vi "UHR-Fleezers Control (host) - Lorentz v3.vi"() -> ()   [LabVIEW 2014] (continued)
  in  "Red FB Gains":T14={"proportional gain (Kc)"=10, "integral gain (Kc*Ts/Ti)"=5, "derivative gain (Kc*Td/Ts)"=0}
  in  "Phase adj. (RI)":i16=20
  out "RI relative phase":i16
  in  "+ phase (RI)":bool
  in  "- phase (RI)":bool
  in  "Blue Laser Modulation Mode":string(combo)
  out "Digital Modulation":bool
  out "Analog Modulation":bool
  out "Laser On":bool
  in  "Get Blue Laser State":bool
  out "Blue laser intensity (V)":dbl
  out "Relative phase (BI AO)":i16
  out "Relative phase (BI DO)":i16
  out "Late Counter (BI DO)":u8
  out "Late Counter (BI AO)":u8
  in  "Initial Phase Adjustment (BI DO)":i16=65
  in  "Initial Phase Adjustment (BI AO)":i16
  in  "Phase adj. (BI AO)":i16=20
  in  "+ phase (BI AO)":bool
  in  "- phase (BI AO)":bool
  in  "Blue int AO ON count adjust":u16=150
  in  "Blue FB Gains":T14={"proportional gain (Kc)"=10, "integral gain (Kc*Ts/Ti)"=5, "derivative gain (Kc*Td/Ts)"=0}
  in  "- phase (BI DO)":bool
  in  "+ phase (BI DO)":bool
  in  "Phase adj. (BI DO)":i16=20
  out "Blue AI Count":u16=600
  in  "Delay (ms)":i32=500
  in  "Send string\nto Blue Laser":bool
  in  "command string":string
  out "command string sent":string="sames 0"
  out "read blue buffer":string
  out "Blue Error Out":errorcluster={"status"=TRUE, "code"=-1073807346, "source"="VISA Write in serial write macro.vi->UHR-Fleezers Control (host) - Lorentz v3.vi"}
  in  "VISA resource name":refnum<visa-resource-name>="Blue-Laser-COM7"
  in  "Blue Laser Modulation\nPower (mW)":string="80"
  in  "Blue Laser Power (mW)\n(Constant Power Mode)":string="70"
  out "Serial Error out":errorcluster={"status"=FALSE, "code"=1073676294, "source"="VISA Read in Arduino input-output.vi->UHR-Fleezers Control (host) - Lorentz v3.vi"}
  in  "PSD Data Period (s)":dbl=0.02 caption="PSD data period (s)" format="%#_6p"
  in  "Flip X Sign":bool=TRUE
  in  "Trap Position FIFO Depth":u32=300000 format="%.0p"
  in  "# Samples/trap":u32=20000
  out "Trap AI Elements/DMA read":u32=320000 format="%.0p"
  out "Ave. Rate (Hz)":dbl=200000.0 format="%#_6p"
  out "FIFO El. Rem.":u32 format="%.0p"
  in  "Phase adj. (AI1)":i16=10
  out "Relative phase (AI1)":i16=-170
  in  "+ phase (AI1)":bool
  in  "- phase (AI1)":bool
  out "Late Counter (AI1)":u8
  in  "Initial Phase Adjustment (AI1)":i16=170
  out "AI rate (Hz)":dbl=200000.0 format="%#_6p"
  in  "AI Count (ticks)":u16=200
  out "# Samples/channel":u32=40000 format="%.0p"
  in  "Trap AI FIFO Depth":u32=900000
  in  "Detector Type":string(combo)="IR-QPD + PSD + FB-QPD X position"
  in  "N Acq Sets (Traps + Fl.)":i16=3
  in  "Sets to FIFO (Traps)":T22={"Set 1"=TRUE, "Set 2"=TRUE, "Set 3"=FALSE}
  in  "FPGA Ave.":dbl=1.0 min=1.0 step=1.0
  out "Ave. Period (s)":dbl=5e-06 format="%#_6p"
  out "DMA Update Period (s)":dbl=0.3
  out "FPGA Averaging":bool
  out "Trap Sets":u32=2
  out "Counts/DMA":dbl=12000000.0 format="%#_6p"
  out "Trap Pos FIFO El Remaining":u32=3 format="%.0p"
  out "Trap Pos Elements/DMA read":u32=200000 format="%.0p"
  out "Trap AI FIFO Timeout":u16=1256
  out "Trap Pos FIFO Timeout":u16=10635
  in  "Serial Settings for arduino":T23={"baud rate"=9600, "data bits"=8, "parity"=enum."None", "stop bits"=10, "flow control"=0, "Time out (ms)"=1000} {"flow control" items=["None"=0, "XON/XOFF"=1, "RTS/CTS"=2, "DTR/DSR"=4]; "stop bits" items=["1.0"=10, "1.5"=15, "2.0"=20]; "data bits" min=5 max=8 step=1; "baud rate" items=["75"=75, "110"=110, "134"=134, "150"=150, "300"=300, "600"=600, "1200"=1200, "1800"=1800, "2400"=2400, "4800"=4800, "7200"=7200, "9600"=9600, "14400"=14400, "19200"=19200, "28800"=28800, "38400"=38400, "56000"=56000, "57600"=57600, "115200"=115200, "128000"=128000, "230400"=230400]}
  in  "VISA resource name":refnum<visa-resource-name>="COM18"
  in  "Serial Error in":errorcluster
  out "error out":errorcluster
  out "error out 2":errorcluster
  in  "Piezo trap 0 position relative to 75 MHz":cluster{"X (V)":dbl, "Y (V)":dbl}={"X (V)"=3.0, "Y (V)"=0.0}
  in  "Piezo Trap Y cal (nm/V)":dbl=200.0
  in  "Piezo Trap X cal (nm/V)":dbl=200.0
  in  "Bottom  1 Harvard Syringe Pump Serial Port":refnum<visa-resource-name>="Bottom-Pump1-COM5"
  in  "Center Harvard Syringe Pump Serial Port":refnum<visa-resource-name>="Central-Pump2-COM6"
  in  "Lost Tether Alarm Threshold (pN)":dbl=0.5
  in  "AOM X Cal (nm/MHz)":dbl=200.0
  in  "MCL X Cal (nm/V)":dbl=739.5
  out "X RF Amplitude Limits (%)":T24={"Minimum"=0.0, "Maximum"=50.0, "Increment"=1.0}
  out "X RF Frequency Limits (MHz)":T24={"Minimum"=60.0, "Maximum"=90.0, "Increment"=1.0}
  out "Y RF Frequency Limits (MHz)":T24={"Minimum"=0.0, "Maximum"=40.0, "Increment"=0.1}
  out "Y RF Amplitude Limits (%)":T24={"Minimum"=0.0, "Maximum"=45.0, "Increment"=1.0}
  in  "Manip. X?":bool=TRUE
  in  "Manip. Y?":bool
  in  "Force Manip Abort":bool
  out "Read cal error":errorcluster={"status"=TRUE, "code"=7, "source"="Open/Create/Replace File in UHR-Fleezers Control (host) - 15.2.1UCBMengV9.vi<APPEND>\nP:\\Data\\160111\\current.cal"}
  in  "DAQ Delay (ms)":u32=1000
  in  "Start Scan":bool
  in  "Scan axis":bool=TRUE
  in  "Osc. amp. (V)":dbl=5.0
  in  "Osc. center (V)":dbl=5.0
  in  "Osc. freq. (Hz) 2":dbl=1.0
  in  "MCL Mode":u16(ring) items=["Manual Positioning", "Sinusoidal Wave", "Linear Scan"]
  in  "Begin (V)":dbl
  in  "End (V)":dbl=10.0
  in  "N Points":dbl=20.0
  in  "Delay to Interlace (s)":dbl
  in  "Delayed Interlace Start":bool
  in  "Read Lateness and Rel Phase":bool=TRUE
  out "Vec Mean of T1 T2":dbl[](array[numeric])=[nan, nan]
  in  "Cal read wait (s)":u32=5
  out "Time tether formed":timestamp=timestamp(3534521622.0325327 s since 1904-01-01)
  in  "Sample Chamber Stage Serial Port":refnum<visa-resource-name>="Sample-Stage-COM1"
  in  "Chemyx Syringe Pump Serial Port":refnum<visa-resource-name>="ASRL3::INSTR"
  in  "Limit Min (MHz)":dbl=10.0 caption="Min (MHz)"
  in  "Limit Max (MHz)":dbl=16.0 caption="Max (MHz)"
  in  "Limits Enable":bool=TRUE caption="Enable"
  out "AI labels":string[](array[string])=["T1 Y", "T1 X", "T1 Sum", "T2 Y", "T2 X", "T2 Sum", "T1 FB X", "T1 FB Sum", "T2 FB X", "T2 FB Sum", "T3 Y", "T3 X", "T3 Sum", "PSD X", "PSD Y", "PSD Sum"]
  in  "Save Trap Pos. Data":bool=TRUE
  in  "Lower Ch. Cap.":bool
  in  "Top 3 Harvard Syringe Pump Serial Port":refnum<visa-resource-name>="Top-Pump3-COM4"
  out "Database link":path=path "C:/Home/Bustamante Lab/Comstock-LabView-Link.udl"
  out "connection reference":T25
  out "FPGA error out":errorcluster
  out "Trigger Signal":dbl[](graph)=[1.953852737276498, 1.8613052147403675]
  in  "Fish mask thresh":dbl=0.5
  in  "Normal (on) or masked test (off)":bool=TRUE
  in  "Stop F (pN) (mask)":dbl=1.0
  in  "Osc. freq. (Hz)":dbl=0.25
  in  "Trap shift\nmethod":bool=TRUE
  in  "Pause rotation":bool
  out "Waveform Chart":dbl(graph)
  in  "Trap 2 phase shift (deg)":dbl caption="Fixed phase shift (deg)"
  in  "Radius (MHz)":dbl=2.0 min=0.0 max=10.0 step=0.1
  out "Trap trajectories":cluster{dbl[], dbl[]}[](graph)
  in  "Move in a Circle":bool
  in  "Center Y Frequency (MHz)":dbl=31.0
  in  "Stop Moving":bool
  in  "2D Motion Frequency (Hz)":dbl=0.25
  in  "2D Motion Trap Separation (MHz)":dbl=0.75 caption="Fixed distance (MHz)" min=0.0 max=10.0 step=0.1
  in  "Time step (ms)":i64=10
  in  "N steps then stop":i32
  in  "Back to start on finish?":bool=TRUE
  in  "Counterclockwise/Clockwise":bool
  out "Trap 1 sum mean":dbl=nan format="%0.2f"
  out "Trap 2 sum mean":dbl=nan format="%0.2f"
  in  "index 1":i32=3
  in  "index 2":i32
  in  "test":bool
  in  "Reset graph":bool
  in  "N steps to plot":i32=1000
  out "Waveform Graph 2":waveform(dbl)(graph)
  in  "Offset 2":dbl
  in  "mult x":dbl
  in  "Offset":dbl
  out "N data samples":dbl
  out "Initial buffer time (s)":dbl
  in  "N initial buffer elements":u16=5000
  in  "Sound ON":bool
  in  "Carrier Frequency (Hz)":dbl=300.0
  in  "number of samples/ch":i32=100000
  in  "sample mode":T26=1 items=["Finite Samples", "Continuous Samples"]
  in  "device ID":u32
  in  "sound format":T27={"sample rate (S/s)"=22050.0, "number of channels"=2, "bits per sample"=16}
  in  "Volume":dbl=1.0 format="%0.2p"
  in  "interpolation mode":u16(ring)=1 items=["coerce", "linear", "spline", "FIR filter"]
  in  "tone or data":bool
  in  "Data channel to sound":i32
  in  "Base N trap periods":u32=50
  in  "Period scale factor":dbl=4.0
  in  "Trap osc amp (MHz)":dbl=1.0
  in  "Osc trap cont.":bool
  in  "Osc traps":bool
  out "Trap OSC Period (s)":dbl=0.003
  out "Writing waveform to fpga memory":bool
  in  "Save trap pos with cal":bool=TRUE
  in  "T1 Osc Enable":bool=TRUE
  in  "T2 Osc Enable":bool=TRUE
  out "DMA remainder":u64
  out "(total save/100) /osc period remainder":u32
  out "Total save/100 remainder":u32
  out "N osc/ (total save/100)":u64=25
  out "N osc / DMA":u64=100
  out "N trap osc periods per save":u64
  out "N trap osc periods per save remainder":u64
  in  "Command":string
  out "Reply":string
  in  "Send Command":bool
  out "Preamp Error Out":errorcluster
  in  "Gain Mode":string(combo)="0"
  in  "Invert Signal":bool
  in  "Sensitivity":string(combo)="0"
  in  "Offset Current Sign":bool=TRUE
  in  "Offset Current Value":string(combo)
  in  "Offset Current":bool
  in  "Bias Voltage":bool
  in  "Bias Voltage (mV)":i32
  in  "Filter Type":string(combo)="4"
  in  "Lowpass 3dB Point":string(combo)="6"
  in  "Highpass 3dB Point":string(combo)
  in  "Filter Reset":bool
  out "Command Sent":string
  out "Gain":string(combo)="0"
  out "Pressure":dbl=0.014364525990046895 format="%#.2f"
  in  "Vacuum":bool=TRUE
  in  "Set zero pressure":bool caption="Vent pressure"
  in  "Laser Control 1":bool
  in  "Laser Control 2":bool
  in  "Laser Control 3":bool
  in  "Laser Control 4":bool
  in  "Laser Control 5":bool
  in  "DAQmx Device Name":tag="Lumicks"
  # "X"
  # "Y"
  # "Data Saving"
  # "External fluorescence triggering tests:"
  # "After"
  # "During"
  # "Trap On?"
  # "BD Flow ON?"
  # "Samp Flow ON?"
  # "Trap Trig. Fl.?"
  # "Zero It"
  # "Floor it\n(e.g., hp unwinding)"
  # "1"
  # "2"
  # "Fl. Down"
  # "Fl. Up"
  # "T1 Y"
  # "T1 X"
  # "T1 Sum"
  # "T2 Y"
  # "T2 X"
  # "T2 Sum"
  # "FB1 X"
  # "FB1 Sum"
  # "FB2 X"
  # "FB2 Sum"
  # "T3 Y"
  # "T3 X"
  # "T3 Sum"
  # "PSD X"
  # "PSD Y"
  # "PSD Sum"
  # "Trap Display:"
  # "APD Display:"
  # "DAQ"
  # "Trap Manipulation"
  # "Bead Calibration"
  # "MCL trap"
  # "Fine Motor Control"
  # "Bottom Pump (#1)"
  # "Central Sample Channels"
  # "Top Pump (#3)"
  # "Rate param is ul/h\nVolume param is ul"
  # "Chemyx Pump 2"
  # "Units: \n1 = ml/m\n2 = ml/h\n3 = ul/m\n4 = ul/h"
  # "Choose method of updating trap RF values: false is usual, true is use external loop method\n(in order to increase possible delay between X and Y signals -- to synchronize X and Y switching)"
  # "Delay to switch frequency and amplitude of boards.\nUsed to align phases of boards (finely)."
  # "X"
  # "Y"
  # "Oscillate Set 1 freq. (debugging)"
  # "BD 1"
  # "BD 2"
  # "Amp switch 1st is disabled in the fpga!\nSeems its also frequency that needs to go first (for all boards tested so far)."
  # "AOD Raster Scan"
  # "Approx. trap separations"
  # "X"
  # "Y"
  # "FPGA\nreading"
  # "DMA\ntransfer"
  # "APD Integration Loop"
  # "APD Gates"
  # "APD 2 (Cy5)"
  # "APD 3 (Cy2)"
  # "APD 1 (Cy3)"
  # "X"
  # "2D"
  # "Y"
  # "1D"
  # "Digital Out Control"
  # "Analog Out Control (Feedback Loop)"
  # "Laser Intensity Analog Input"
  # "Operational note:\n\nUse the digital out control to adjust red laser\ntiming (fine tuning).\n\nAt the moment, the red laser analog out\ncontrol timing is identical and set by green \nlaser AO timing (in the same loop).  Otherwise\nyou can not get synchronous timing with the\ncurrent AO expansion board.\n\nSimilarly, the AI measurement is also \nsimultaneous for all three lasers (for the same\nreason).\n\nThese controls are kept for possible future\nuse."
  # "Analog Out Control (Feedback Loop)"
  # "Digital Out Control"
  # "Laser Intensity Analog Input"
  # "Operational note:\n\nThe AI measurement is simultaneous for all three lasers\n(see red laser note).\n\nThese controls are kept for possible future use."
  # "Analog Out Control (Feedback Loop)"
  # "Laser Intensity Analog Input"
  # "Digital Out Control"
  # "Total AI Rates (NOT rates/trap)"
  # "(Samples/trap x Trap Sets)"
  # "(Samples/channel x\n8 if averaging (8 channels)\n4 if no averaging)"
  # "Trap 1"
  # "Trap 2"
  # "Flour./Trap 3"
  # "External Video Window"
  # "3: IR LED\n2: Blue LED"
  # "MCL Position Debugging"
  # "Temporary Control Storage\n(these used to be somewhere else, still want to keep them)"
  # "Database config"
  # "Y"
  # "X"
  # "Trap Position Difference Limits"
  # "Start trapping above center (> center MHz)\n\nNegative trap separation means trap 2 follows\n(starts to the right)"
  # "Initialization"
  # "Radius initially determined by center\nand current location (then can be changed)"
  # "Active (oscillating) trap calibration:"
  # "All these remainders\nshould be 0."
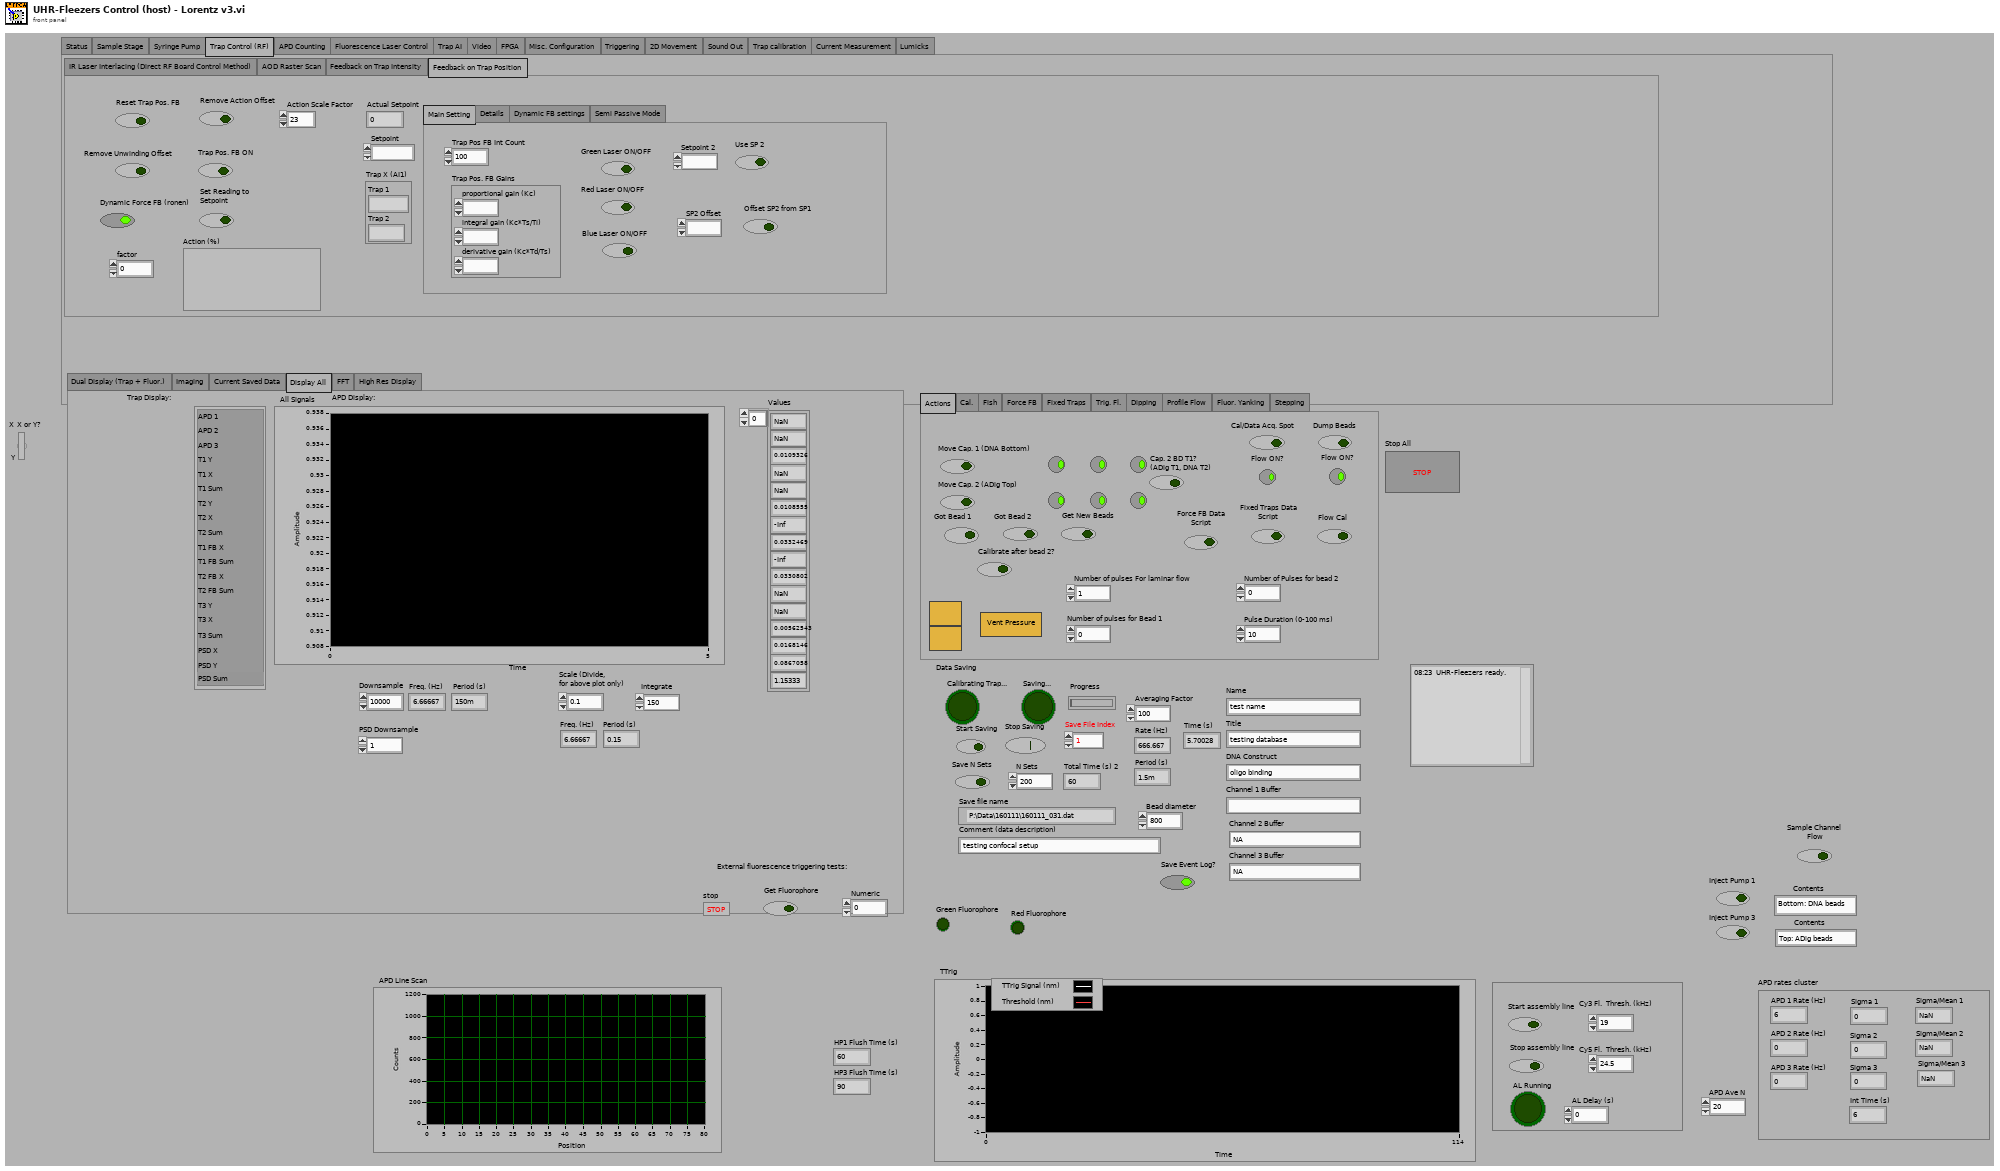
[diagram p1: front panel]
types:
  T1 = cluster{"APD 1 Rate (Hz)":dbl, "APD 2 Rate (Hz)":dbl, "APD 3 Rate (Hz)":dbl, "Sigma/Mean 1":dbl, "Int Time (s)":dbl, "Sigma 1":dbl, "Sigma 2":dbl, "Sigma 3":dbl, "Sigma/Mean 2":dbl, "Sigma/Mean 3":dbl}
  T2 = enum32{"Actions", "Cal.", "Fish", "Force FB", "Fixed Traps", "Trig. Fl.", "Dipping", "Profile Flow", "Fluor. Yanking", "Stepping"}
  T3 = enum32{"Dual Display (Trap + Fluor.)", "Imaging", "Current Saved Data", "Display All", "FFT", "High Res Display"}
  T4 = cluster{"T1 X":dbl, "T2 X":dbl, "T3 X":dbl, "T3 Y":dbl}
  T5 = cluster{"T1 X":bool, "T2 X":bool, "T3 X":bool, "T3 Y":bool}
  T6 = typedef "IMAQ Image.ctl" = refnum<image>
  T7 = enum32{"Status", "Sample Stage", "Syringe Pump", "Trap Control (RF)", "APD Counting", "Fluorescence Laser Control", "Trap AI", "Video", "FPGA", "Misc. Configuration", "Triggering", "2D Movement", "Sound Out", "Trap calibration", "Current Measurement", "Lumicks"}
  T8 = cluster{"T2 alpha_x (nm/V)":dbl, "T2 offset_x (mV)":dbl, "T2 kappa_x (pN/nm)":dbl}
  T9 = cluster{"T1 alpha_x (nm/V)":dbl, "T1 offset_x (mV)":dbl, "T1 kappa_x (pN/nm)":dbl}
  T10 = cluster{"Pump 1":cluster{"Diameter (mm)":dbl, "Units":dbl, "Volume":dbl, "Rate":dbl}, "Pump 2":cluster{"Diameter (mm)":dbl, "Units":dbl, "Volume":dbl, "Rate":dbl}, "Pump 3":cluster{"Diameter (mm)":dbl, "Units":dbl, "Volume":dbl, "Rate":dbl}}
  T11 = enum32{"IR Laser Interlacing (Direct RF Board Control Method)", "AOD Raster Scan", "Feedback on Trap Intensity", "Feedback on Trap Position"}
  T12 = typedef "LVPoint32TypeDef.ctl" = cluster{"Horizontal":i32, "Vertical":i32}
  T13 = cluster{"Scan Range AOD (nm) 2":dbl, "Step Size AOD (nm) 2":dbl, "Scan Speed AOD (nm/s) 2":dbl, "Number of scans (AOD) 2":u16, "Label":string}[]
  T14 = cluster{"proportional gain (Kc)":i16, "integral gain (Kc*Ts/Ti)":i16, "derivative gain (Kc*Td/Ts)":i16}
  T15 = cluster{"Trap 1":fxp<+/-,16,1>, "Trap 2":fxp<+/-,16,1>}
  T16 = enum32{"Main Setting", "Details", "Dynamic FB settings", "Semi Passive Mode"}
  T17 = cluster{"proportional gain (Kc)":fxp<+/-,16,8>, "integral gain (Kc*Ts/Ti)":fxp<+/-,16,8>, "derivative gain (Kc*Td/Ts)":fxp<+/-,16,8>}
  T18 = cluster{"output high":fxp<+/-,16,1>, "output low":fxp<+/-,16,1>}
  T19 = cluster{"Set 1":fxp<+/-,16,1>, "Set 2":fxp<+/-,16,1>}
  T20 = cluster{"Trap 1X offset":dbl[], "Trap 2X offset":dbl[]}
  T21 = enum32{"Main Controls", "Green laser (532 nm)", "Red laser (633 nm)", "Blue laser (473 nm)"}
  T22 = cluster{"Set 1":bool, "Set 2":bool, "Set 3":bool}
  T23 = cluster{"baud rate":u32, "data bits":u16, "parity":enum16{"None", "Odd", "Even", "Mark", "Space"}, "stop bits":u16, "flow control":u16, "Time out (ms)":u32}
  T24 = typedef "LVMinMaxIncTypeDef.ctl" = cluster{"Minimum":dbl, "Maximum":dbl, "Increment":dbl}
  T25 = typedef "NI_Database_API.lvlib/Conn ObjectReference.ctl" = refnum<k1>
  T26 = typedef "Sampling Mode.ctl" = i32
  T27 = typedef "Sound Data Format.ctl" = cluster{"sample rate (S/s)":dbl, "number of channels":i32, "bits per sample":i32}
  T28 = typedef "nirio_resource_hc.ctl" = tag
  T29 = typedef "Image Type" = u32
  T30 = typedef "Pressure Control.lvclass/Pressure Control Config.ctl" = cluster{"daqmx_channel":string, "terminal_configuration":string}
  T31 = cluster{string, "TTL line # Pressure Up":u8, bool, bool}
  T32 = cluster{string, "TTL line # Pressure Down":u8, bool, bool}
  T33 = cluster{string, "TTL line # Pressure Vacuum":u8, bool, bool}
  T34 = cluster{string, "TTL line # Pressure Vacuum":u8, bool, bool}[]
  T35 = cluster{"New Image":T6, "New Image":T6, "New Image":T6, "New Image":T6, "New Image":T6}
  T36 = typedef "openfpgaref.8.6.ctl" = refnum<k20>
  T37 = typedef "XDNodeRunTimeDep.lvlib/timing_clust.ctl" = cluster{"Expected End [f-1]":u64, "Actual End [f-1]":u64, "Finished Late? [f-1]":bool, "Expected End [i-1]":u64, "Actual End [i-1]":u64, "Finished Late? [i-1]":bool, "Expected Start [i]":u64, "Actual Start [i]":u64, "Expected Start [f]":u64, "Actual Start [f]":u64, "Source Name":string, "Structure Name":string, "Period":i64, "Deadline":i64, "Offset":i64, "Start":i64, "Priority":i32, "Timeout":i32, "Mode":T38, "Wakeup Reason":T39, "Error":errorcluster, "Source Type":string, "Secondary Source Type":string, "Global End Time":u64, "Global Start Time":u64, "Frame Duration":u64, "Iteration Duration":u64, "Assigned CPU":i32, "I/O Scan Engine Mode":u32}
  T38 = typedef "XDNodeRunTimeDep.lvlib/nitl_modes.ctl" = enum32{"No Change", "Process missed periods, maintain original phase", "Discard missed periods, maintain original phase", "Process missed periods, ignore original phase", "Discard missed periods, ignore original phase"}
  T39 = typedef "XDNodeRunTimeDep.lvlib/wakeup.ctl" = enum32{"Normal", "Aborted", "Asynchronous wakeup", "Timing source error", "Timed loop error", "Timeout"}
  T40 = enum32{"Status", "Sample Stage", "Syringe Pump", "Trap Control (RF)", "APD Counting", "Fluorescence Laser Control", "Trap AI", "Video", "FPGA"}
  T41 = enum32{"Status", "Sample Stage", "Syringe Pump", "Trap Control (RF)", "APD Counting", "Fluorescence Laser Control", "Trap AI", "Video", "FPGA", "Misc. Configuration"}
  T42 = enum16{"CONNECT", "INITIALIZE VALVES", "DISCONNECT", "MOVE VALVE"}
  T43 = enum16{"empty", "write", "read oldest (queue)", "read newest (stack)", "read all"}
  T44 = enum16{"open", "replace", "create", "open or create", "replace or create", "replace or create with confirmation"}
  T45 = enum16{"big-endian, network order", "native, host order", "little-endian"}
  T46 = cluster{"Scan Range AOD (nm) 2":dbl, "Step Size AOD (nm) 2":dbl, "Scan Speed AOD (nm/s) 2":dbl, "Number of scans (AOD) 2":u16, "Label":string}
  T47 = cluster{"[0]":dbl, "[1]":dbl, "[2]":dbl, "[3]":dbl, "[4]":dbl, "[5]":dbl}
  T48 = cluster{"Diameter (mm)":dbl, "Units":dbl, "Volume":dbl, "Rate":dbl}
  T49 = cluster{"Left":void, "Top":void, "Width":void, "Height":void}
  T50 = cluster{cluster{"Left":void, "Top":void, "Width":void, "Height":void}}[]
  T51 = typedef "Sound Output Task ID.ctl" = u32
  T52 = enum32{"Normal Display", "Dual Display (APD)", "FFT", "High Res Display"}
  T53 = cluster{"Origin Pixel":cluster{"X":sgl, "Y":sgl}, "Angle Relative to Horizontal (deg)":sgl, "Axis Reference":u32}
  T54 = typedef "Simple Grid Descriptor" = cluster{"X Step":sgl, "Y Step":sgl, "Unit":T55}
  T55 = typedef "Image Unit" = enum32{"Undefined", "Angström", "Micrometer", "Millimeter", "Centimeter", "Meter", "Kilometer", "Microinch", "Inch", "Feet", "Nautical miles", "Standard miles", "Steps"}
  T56 = cluster{"averaging mode":u16, "weighting mode":u16, "number of averages":u32}
  T57 = cluster{"dB On (F)":bool, "unwrap phase (F)":bool, "convert to degree (F)":bool}
  T58 = cluster{"Scan Range (nm)":dbl, "MCL Step Position Ratio":dbl, "MCL/AOM Scale Tweak":dbl, "MCL X Cal (nm/V)":dbl, "MCL Step Increment (V_int)":dbl, "Total Counts (ticks)":u16, "Scan steps (AOD)":u64, "Cycles/step (AOD)":u64}
  T59 = cluster{"Actual MCL Inc (V)":dbl, "Scan steps (MCL)":u64, "Scan lines (y)":u64, "AO1":dbl, "AO2":dbl}
  T60 = cluster{"APD 1":u32[], "APD 2":u32[], "APD 3":u32[]}
  T61 = cluster{"RMS[0]":dbl, "RMS[1]":dbl, "RMS[2]":dbl, "RMS[3]":dbl}
  T62 = cluster{"Mean [0]":dbl, "Mean [1]":dbl, "Mean [2]":dbl, "Mean [3]":dbl}
  T63 = cluster{"f0":dbl, "df":dbl, "magnitude":dbl[]}[][]
  T64 = cluster{"Comment (data description)":string, "Channel 1 Buffer":string, "Channel 2 Buffer":string, "Channel 3 Buffer":string, "Title":string, "DNA Construct":string, "Bead diameter":dbl, "Name":string}
diagram:
  w7 = 90.0
  w35 = T29 2 items=["Grayscale (U8)", "Grayscale (I16)", "Grayscale (SGL)", "Complex (CSG)", "RGB (U32)", "HSL (U32)", "RGB (U64)", "Grayscale (U16)"] ("Image Type")
  # "X limits"
  # "Amp Lmits"
  # "Freq Limits"
  # "Changed by Ronen - All events relating to activation of the pumps have been disabled: 56, 55, 54, 53, 52, 51, 50, 49, 48, 47, 46, 45, 44, 43, 41, 40"
  # "Harvard Pump control disabled by Hendrik"
  # "Settings to help prevent AOM/D damage"
  # "Initialize the FPGA DAQ card itself"
  # "Reset the DAQ card."
  # "Specify the DAQ card and the FPGA code to run"
  # "Bottom 1 Harvard"
  # "Top 3 Harvard"
  # "Center Harvard"
  n1 = disable-structure shown="Enabled" {
    frame Enabled {
      w105 = FALSE
      # "This Control added by\nRonen to enable direct\nControl of pressure pulse\nlength to enable fine flow\ncontrol"
      # "Start out with all lines set to zero"
      n2 = Format Into String(format string="%s/port0/line5:1, %s/port1/line0:3", "DAQmx Device Name", "DAQmx Device Name") -> (resulting string=w97:string)  [unwired: 2 in, 1 out]
      n3 = Format Into String(format string="%s/ai0", "DAQmx Device Name") -> (resulting string=w95:string)  [unwired: 2 in, 1 out]
      n4 = In Range and Coerce(upper limit=100.0, x="Pulse Duration (0-100 ms)", lower limit=0.0) -> (coerced(x)=w80:dbl)  [unwired: 1 out]
      n5 = Bundle By Name(cluster=T30 {"daqmx_channel"="", "terminal_configuration"=""} ("Pressure Control Config"), "daqmx_channel"=w95, "terminal_configuration"="RSE") -> (w112:T30)
      n6 = To Unsigned Long Integer(number=w80) -> (unsigned 32bit integer=w79:u32)
      n7 = Bundle("Pressure up", "TTL line # Pressure Up"=u8 6, w105, w105) -> (w103:T31)  [unwired: 1 in]
      n8 = Bundle("Pressure down", "TTL line # Pressure Down"=u8 8, w105, w105) -> (w104:T32)  [unwired: 1 in]
      n9 = Bundle("Pressure vacuum", "TTL line # Pressure Vacuum"=u8 7, w105, w105) -> (w102:T33)  [unwired: 1 in]
      n10 = Build Array(w103, w104, w102) -> (w101:T34)
      n11 = call "Initialize.vi"("Pulse duration (ms)"=w79, "TTL Ports"=w97, "TTL in"=refnum<class "TTL.lvclass"> refnum ("TTL.lvclass")) -> ("error out"=w100:errorcluster, "TTL out"=w89:refnum<class "TTL.lvclass">)  [unwired: 7 in]
      n12 = call "Initialize.vi"("TTL Lines"=w101, "error in (no error)"=w100, "TTL"=w89, "Pressure Control Config"=w112, "Pressure Control in"=refnum<class "Pressure Control.lvclass"> refnum ("Pressure Control.lvclass")) -> ("error out"=w117:errorcluster, "Pressure Control out"=w99:refnum<class "Pressure Control.lvclass">)  [unwired: 5 in]
      n13 = call "Get line states.vi"("error in (no error)"=w117, "TTL in"=w89) -> ("error out"=w84:errorcluster, "Current line states"=w85:bool[], "TTL out"=w88:refnum<class "TTL.lvclass">)  [unwired: 7 in]
      n14 = Array Size(array=w85) -> (size(s)=w86:i32)
      n15 = for {
        N: w86 -> [_]
        shift-right: [w123] -> w87
        shift-left: w88 -> [w124]
        shift-right: [w121] -> w118
        shift-left: w84 -> [w122]
        i -> [w120]
        n16 = call "Set line.vi"("error in (no error)"=w122, "Action"=enum16{"Open", "Close", "Toggle"}."Open", "Line number"=w120, "TTL in"=w124) -> ("error out"=w121:errorcluster, "TTL out"=w123:refnum<class "TTL.lvclass">)  [unwired: 6 in]
      }
      n17 = case shown="No Error" w118 {
        selector: w118 -> [_ w208]
        tunnel: w99 -> [w129 _]
        tunnel: w87 -> [w128 _]
        tunnel: [w125 w207] -> w92
        frame No Error {
          n18 = while {
            shift-right: [w137] -> w126
            shift-left: w129 -> [w136]
            shift-right: [w135] -> w127
            shift-left: w128 -> [w134]
            stop <- w132 stop-if-true
            n19 = call "Get pressure.vi"("Pressure Control in"=w136) -> ("Pressure"=→"Pressure":dbl)  [unwired: 7 in, 3 out]
            n20 = event shown="[0] Timeout" {
              selector: _ -> [_ _ _ _ _ _ _ _ _ _ _ _ _]
              dyn-events: _ -> [_ _ _ _ _ _ _ _ _ _ _ _ _]
              timeout: 100 -> [_ _ _ _ _ _ _ _ _ _ _ _ _]
              tunnel: [w140 w143 w144 w149 w153 w158 w163 w175 w182 w188 w194 w200 w206] -> w137
              tunnel: w136 -> [w140 w143 w145 w150 w154 w159 w164 w176 w182 w188 w194 w200 w206]
              tunnel: [w139 w142 w146 w151 w155 w160 w165 w173 w180 w186 w192 w198 w204] -> w135
              tunnel: w134 -> [w139 w142 w146 w151 w155 w160 w165 w174 w181 w187 w193 w199 w205]
              tunnel: [_ TRUE _ _ _ _ _ _ _ _ _ _ _] -> w132
              tunnel: [_ _ w147 w152 w156 w161 w166 w172 w177 w183 w189 w195 w201] -> w131
              event Timeout {
                n21 = event-data() -> ()  [unwired: 1 in, 2 out]
              }
              event "Stop All": Value Change {
                n22 = event-data() -> ()  [unwired: 1 in, 6 out]
              }
              event "Vent pressure": Value Change {
                n23 = event-data() -> ()  [unwired: 1 in, 5 out]
                n24 = call "Vent.vi"("Pressure Control in"=w145) -> ("error out"=w147:errorcluster, "Pressure Control out"=w144:refnum<class "Pressure Control.lvclass">)  [unwired: 9 in]
              }
              event "Vacuum": Value Change {
                n25 = event-data() -> ("NewVal"=w148:bool)  [unwired: 1 in, 4 out]
                n26 = call "Set vacuum.vi"("Vacuum?"=w148, "Pressure Control in"=w150) -> ("error out"=w152:errorcluster, "Pressure Control out"=w149:refnum<class "Pressure Control.lvclass">)  [unwired: 8 in]
              }
              event "Set zero pressure": Value Change {
                n27 = event-data() -> ()  [unwired: 1 in, 5 out]
                n28 = call "Set zero pressure to current pressure.vi"("Pressure Control in"=w154) -> ("error out"=w156:errorcluster, "Pressure Control out"=w153:refnum<class "Pressure Control.lvclass">)  [unwired: 8 in, 1 out]
              }
              event "Pressure Up": Value Change {
                n29 = event-data() -> ()  [unwired: 1 in, 5 out]
                n30 = call "Pressure pulse.vi"("Up or down?"=enum16{"Up", "Down"}."Up", "Pressure Control in"=w159) -> ("error out"=w161:errorcluster, "Pressure Control out"=w158:refnum<class "Pressure Control.lvclass">)  [unwired: 8 in]
              }
              event "Pressure Down": Value Change {
                n31 = event-data() -> ()  [unwired: 1 in, 5 out]
                n32 = call "Pressure pulse.vi"("Up or down?"=enum16{"Up", "Down"}."Down", "Pressure Control in"=w164) -> ("error out"=w166:errorcluster, "Pressure Control out"=w163:refnum<class "Pressure Control.lvclass">)  [unwired: 8 in]
              }
              event "Pulse Duration (0-100 ms)": Value Change {
                # "Event added by Ronen to allow for changes\nin pulse duration as program is running"
                n33 = event-data() -> ()  [unwired: 1 in, 6 out]
                n34 = local read "Pulse Duration (0-100 ms)"() -> (w170:dbl)
                n35 = In Range and Coerce(upper limit=100.0, x=w170, lower limit=0.0) -> (coerced(x)=w168:dbl)  [unwired: 1 out]
                n36 = To Unsigned Long Integer(number=w168) -> (unsigned 32bit integer=w167:u32)
                n37 = call "Change TTL - Ronen.vi"("Pulse Duration (ms)"=w167, "TTL.lvclass"=w174) -> ("error out"=w172:errorcluster, "TTL.lvclass"=w173:refnum<class "TTL.lvclass">)  [unwired: 8 in]
                n38 = call "Update TTL - Ronen.vi"("TTL.lvclass"=w173, "Pressure Control in"=w176) -> ("Pressure Control out"=w175:refnum<class "Pressure Control.lvclass">)  [unwired: 8 in, 1 out]
              }
              event "Laser Control 1": Value Change {
                n39 = event-data() -> ()  [unwired: 1 in, 5 out]
                n40 = call "Set line.vi"("Action"=enum16{"Open", "Close", "Toggle"}."Toggle", "Line number"=u8 0, "TTL in"=w181) -> ("error out"=w177:errorcluster, "TTL out"=w180:refnum<class "TTL.lvclass">)  [unwired: 7 in]
              }
              event "Laser Control 2": Value Change {
                n41 = event-data() -> ()  [unwired: 1 in, 5 out]
                n42 = call "Set line.vi"("Action"=enum16{"Open", "Close", "Toggle"}."Toggle", "Line number"=u8 1, "TTL in"=w187) -> ("error out"=w183:errorcluster, "TTL out"=w186:refnum<class "TTL.lvclass">)  [unwired: 7 in]
              }
              event "Laser Control 3": Value Change {
                n43 = event-data() -> ()  [unwired: 1 in, 5 out]
                n44 = call "Set line.vi"("Action"=enum16{"Open", "Close", "Toggle"}."Toggle", "Line number"=u8 2, "TTL in"=w193) -> ("error out"=w189:errorcluster, "TTL out"=w192:refnum<class "TTL.lvclass">)  [unwired: 7 in]
              }
              event "Laser Control 4": Value Change {
                n45 = event-data() -> ()  [unwired: 1 in, 5 out]
                n46 = call "Set line.vi"("Action"=enum16{"Open", "Close", "Toggle"}."Toggle", "Line number"=u8 3, "TTL in"=w199) -> ("error out"=w195:errorcluster, "TTL out"=w198:refnum<class "TTL.lvclass">)  [unwired: 7 in]
              }
              event "Laser Control 5": Value Change {
                n47 = event-data() -> ()  [unwired: 1 in, 5 out]
                n48 = call "Set line.vi"("Action"=enum16{"Open", "Close", "Toggle"}."Toggle", "Line number"=u8 4, "TTL in"=w205) -> ("error out"=w201:errorcluster, "TTL out"=w204:refnum<class "TTL.lvclass">)  [unwired: 7 in]
              }
            }
            n49 = call <vilib>:"Simple Error Handler.vi"("error in (no error)"=w131) -> ()  [unwired: 4 in, 5 out]
          }
          n50 = call "Close.vi"("Pressure Control in"=w126) -> ("error out"=w130:errorcluster)  [unwired: 9 in, 1 out]
          n51 = call "Close.vi"("error in (no error)"=w130, "TTL in"=w127) -> ("error out"=w125:errorcluster)  [unwired: 8 in, 1 out]
        }
        frame Error {
          n52 = call <vilib>:"Simple Error Handler.vi"("error in (no error)"=w208) -> ("error out"=w207:errorcluster)  [unwired: 4 in, 4 out]
        }
      }
      n53 = property on="DAQmx Device Name" class="DAQmxName"("Visible"=FALSE) -> ()  [unwired: 2 in, 2 out]
      n54 = call <vilib>:"Clear Errors.vi"("error in (no error)"=w92) -> ("error out"=w90:errorcluster)  [unwired: 5 in, 1 out]
      n55 = property on="DAQmx Device Name" class="DAQmxName"(error in=w90, "Visible"=TRUE) -> ()  [unwired: 1 in, 2 out]
    }
    frame Disabled {
    }
  }
  n56 = disable-structure shown="Disabled" {
    disable-tunnel: [w240 _] -> w58
    disable-tunnel: [w237 _] -> w47
    disable-tunnel: [w236 _] -> w46
    disable-tunnel: [w231 _] -> w42
    disable-tunnel: [w230 _] -> w41
    disable-tunnel: [w229 _] -> w40
    disable-tunnel: [w228 _] -> w39
    disable-tunnel: [w225 _] -> w31
    disable-tunnel: [w220 _] -> w12
    disable-tunnel: [w213 _] -> w11
    disable-tunnel: [w210 _] -> w10
    frame Disabled {
      w212 = u16 20 items=["1.0"=10, "1.5"=15, "2.0"=20] ("stop bits (10: 1 bit)")
      w223 = u16 20 items=["1.0"=10, "1.5"=15, "2.0"=20] ("stop bits (10: 1 bit)")
      w226 = u16 10 items=["1.0"=10, "1.5"=15, "2.0"=20] ("stop bits (10: 1 bit)")
      w232 = u16 20 items=["1.0"=10, "1.5"=15, "2.0"=20] ("stop bits (10: 1 bit)")
      w234 = u16 20 items=["1.0"=10, "1.5"=15, "2.0"=20] ("stop bits (10: 1 bit)")
      w238 = u16 20 items=["1.0"=10, "1.5"=15, "2.0"=20] ("stop bits (10: 1 bit)")
      # "Bottom 1 Harvard"
      # "Top 3 Harvard"
      # "Center Harvard"
      n57 = call-poly "VISA Configure Serial Port"("VISA resource name"=refnum<visa-resource-name> "COM2", "baud rate (9600)"=u32 9600, "stop bits (10: 1 bit)"=w223) -> ("VISA resource name out"=w213:refnum<visa-resource-name>, "error out"=→"Preamp Error Out":errorcluster)  [unwired: 4 in, 7 out]
      n58 = call-poly "VISA Configure Serial Port"("VISA resource name"=refnum<visa-resource-name> "COM2", "baud rate (9600)"=u32 9600, "stop bits (10: 1 bit)"=w212) -> ("VISA resource name out"=w210:refnum<visa-resource-name>)  [unwired: 4 in, 8 out]
